vi "VisualizePPS2.vi"() -> ()   [LabVIEW 2018, in "Visualization.lvlib" / "VisualizeAcPwr.lvclass"]
uses:
  VisualizeAcPwr.lvclass
  <vilib>/event_ctls.llb/usereventprio.ctl
  VisualizeBase/VisualizeBase_class/Requests/clUserEventType.ctl
  <vilib>/Utility/error.llb/Error Cluster From Error Code.vi
  <vilib>/ErrorRing/Error Ring.xnode
  VisualizeBase/VisualizeBase_class/VisualizeBase.lvclass
  <userlib>/NIST/NISTErrorLib/NISTErrorLib.lvlib
  AcPwr/AcPwrModule/AcPwrModule.lvlib
panel:
  out "Incorrect DataType?":bool
  in  "PluginName":string="AcPwr.PPS2"
  out "PacificPower":waveform(dbl)[](graph)=[{"t0"=timestamp(3657294743.1094904 s since 1904-01-01), "dt"=1.0, "Y"=[46.242]}, {"t0"=timestamp(3657294743.1094904 s since 1904-01-01), "dt"=1.0, "Y"=[0.304]}, {"t0"=timestamp(3657294743.1094904 s since 1904-01-01), "dt"=1.0, "Y"=[60.0]}] caption="4140002"
  in  "btnStop":bool
  in  "btnReset":bool
  in  "btnClear":bool
  out "ErrorArray":errorcluster[](array[cluster])
  in  "PlotYAxis":u32[](array[numeric])=[0, 1, 0, 0] max=1
  in  "QueueName":string="PPSVQ"
  # "0=Left Axis and 1=Right Axis"
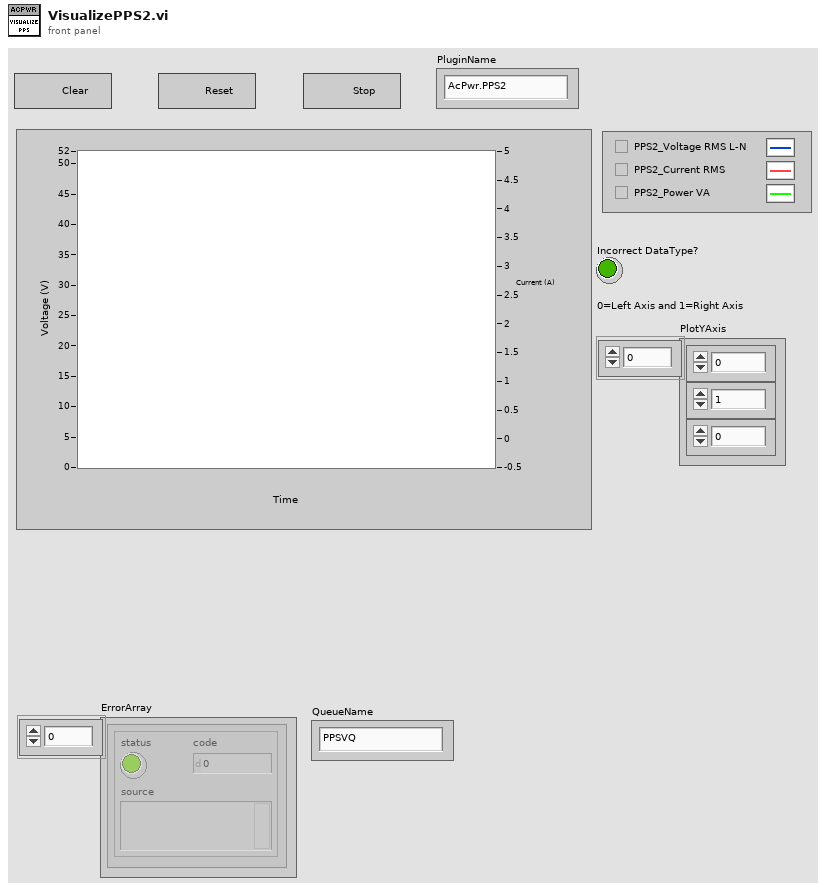
[diagram p1: front panel]
types:
  T1 = typedef "Visualization.lvlib/VisualizeBase.lvclass/clRequestEvents.ctl" = cluster{"StopRequest":refnum<user-event>, "ResetRequest":refnum<user-event>}
  T2 = typedef "AcPwrModule.lvlib/clBroadcastEvents.ctl" = cluster{"DidInit":refnum<user-event>, "StatusUpdate":refnum<user-event>, "ErrorReport":refnum<user-event>, "DidStop":refnum<user-event>, "PathToINI":refnum<user-event>, "Measurements":refnum<user-event>, "LoadConfigFile":refnum<user-event>, "GetSettings":refnum<user-event>, "SetSettings":refnum<user-event>, "GetType&ID":refnum<user-event>, "GotSettings":refnum<user-event>}
  T3 = typedef "Visualization.lvlib/VisualizeBase.lvclass/clUserEventType.ctl" = cluster{"BusIndex":i8, "Data":variant}
  T4 = typedef "usereventprio.ctl" = enum32{"high priority", "normal priority"}
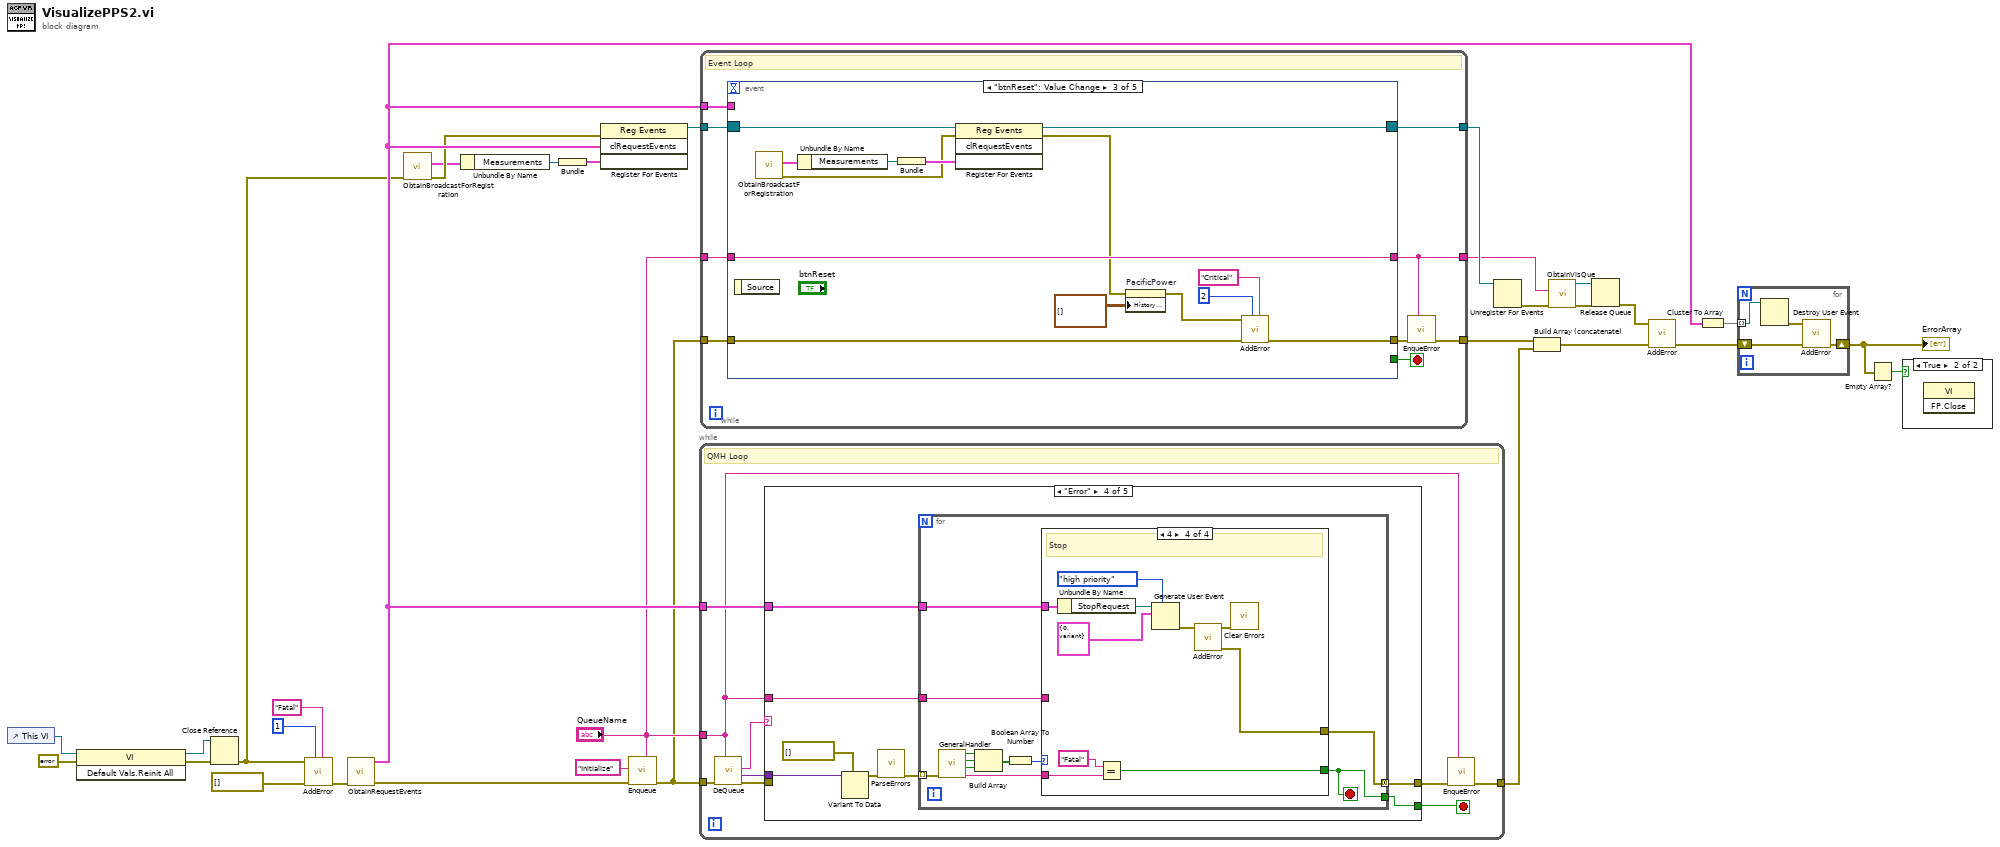
[diagram p0: block diagram]
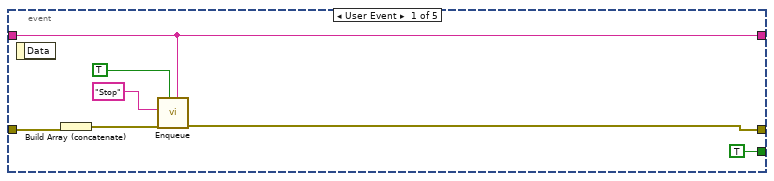
[diagram p2: hidden frame]
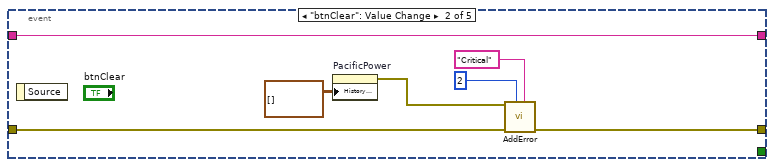
[diagram p3: hidden frame]
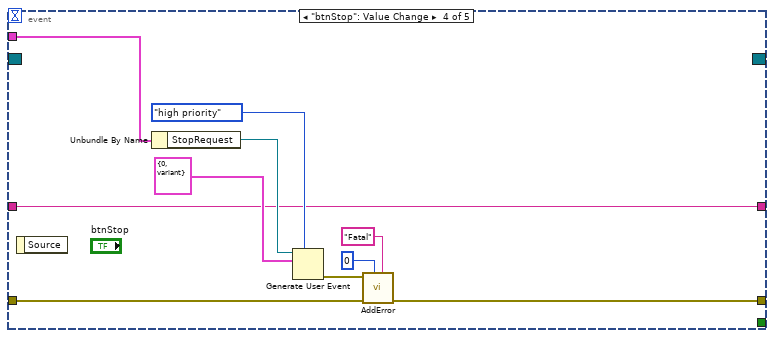
[diagram p4: hidden frame]
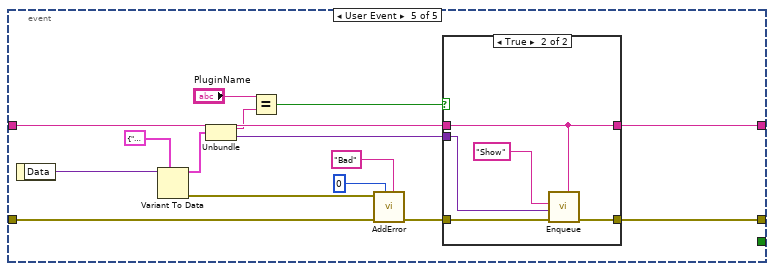
[diagram p5: hidden frame]
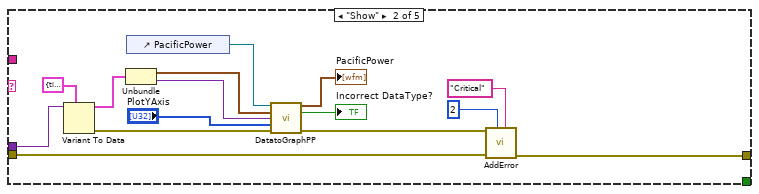
[diagram p8: hidden frame]
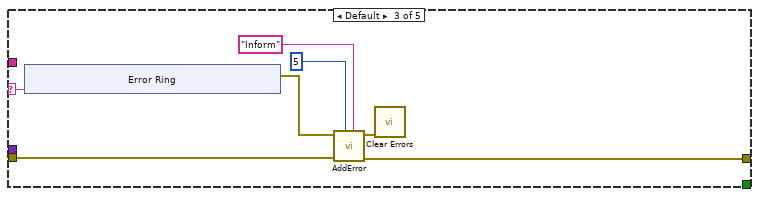
[diagram p9: hidden frame]
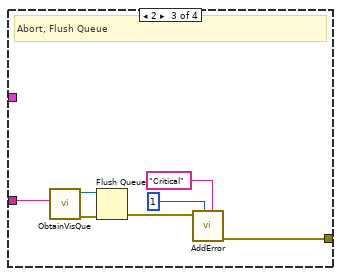
[diagram p12: hidden frame]
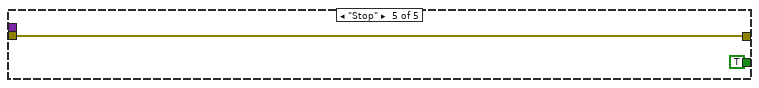
[diagram p13: hidden frame]
diagram:
  n1 = control-ref of="This VI"() -> (w14:refnum<vi>)
  n2 = invoke class="VI" method="Default Vals.Reinit All"(reference=w14, error in=errorcluster {"status"=FALSE, "code"=0, "source"=""} ("error in (no error)")) -> (reference out=w11:refnum<vi>, error out=w12:errorcluster)  [unwired: 1 in, 1 out]
  n3 = Close Reference(reference=w11, error in (no error)=w12) -> (error out=w10:errorcluster)
  n4 = call <userlib>:"AddError.vi"("Severity"="Fatal" ("String"), "Priority"=u8 1, "ErrorArray"=errorcluster[] [], "error in (no error)"=w10) -> ("ErrorArray"=w30:errorcluster[])  [unwired: 6 in, 1 out]
  n5 = call "ObtainRequestEvents.vi"("Error"=w30) -> ("Error"=w15:errorcluster[], "clRequestEvents"=w19:T1)  [unwired: 9 in]
  n6 = call "ObtainBroadcastForRegistration.vi"("error in (no error)"=w10) -> ("error out"=w9:errorcluster, "clBroadcastEvents"=w8:T2)  [unwired: 9 in]
  n7 = Unbundle By Name(w8) -> ("Measurements"=w17:refnum<user-event>)
  n8 = Bundle("Measurements"=w17) -> (w16:cluster{"Measurements":refnum<user-event>})  [unwired: 1 in]
  n9 = register-events(error in=w9, w19, w16) -> (reference out=w31:refnum<event-registration>)  [unwired: 1 in, 1 out]
  n10 = call "Enqueue.vi"("QueName"="QueueName", "Error"=w15, "Message"="Initialize") -> ("Error"=w2:errorcluster[])  [unwired: 8 in]
  n11 = while {
    tunnel: w2 -> [w41]
    tunnel: [w35] -> w26
    tunnel: "QueueName" -> [w33]
    tunnel: w19 -> [w34]
    stop <- w36 stop-if-true
    # "QMH Loop"
    n12 = call "DeQueue.vi"("QueName"=w33, "Error"=w41) -> ("Error"=w38:errorcluster[], "Data"=w39:variant, "Message"=w40:string)  [unwired: 7 in]
    n13 = case shown="\"Error\"" w40 {
      selector: w40 -> [_ _ w64 _ _]
      tunnel: w39 -> [_ w55 _ w79 _]
      tunnel: w38 -> [w42 w52 w62 _ w108]
      tunnel: [w42 w57 w61 w75 w108] -> w37
      tunnel: [_ _ _ w74 TRUE] -> w36
      tunnel: w34 -> [_ _ _ w73 _]
      tunnel: w33 -> [_ _ _ w72 _]
      frame "Initialize" {
      }
      frame "Show" {
        n14 = Variant To Data(type=cluster{timestamp, "Data":variant} {timestamp(0 s since 1904-01-01), "Data"=variant}, Variant=w55) -> (data=w56:cluster{timestamp, "Data":variant}, error out=w47:errorcluster)  [unwired: 1 in]
        n15 = Unbundle(w56) -> (w44:timestamp, "Data"=w43:variant)
        n16 = control-ref of="PacificPower"() -> (w48:refnum<vi>)
        n17 = call "DatatoGraphPP.vi"("PacificPowerChartReference"=w48, "Current time"=w44, "Data"=w43, "PlotYAxis"="PlotYAxis", "error in (no error)"=w47) -> ("Array"=→"PacificPower":waveform(dbl)[], "Incorrect DataType?"=→"Incorrect DataType?":bool, "error out"=w50:errorcluster)  [unwired: 8 in]
        n18 = call <userlib>:"AddError.vi"("Severity"="Critical" ("String"), "Priority"=u8 2, "ErrorArray"=w52, "error in (no error)"=w50) -> ("ErrorArray"=w57:errorcluster[])  [unwired: 6 in, 1 out]
      }
      frame Default {
        n19 = xnode "Error Ring"("parameter 0"=w64) -> ("error out"=w63:errorcluster)
        n20 = call <userlib>:"AddError.vi"("Severity"="Inform" ("String"), "Priority"=u8 5, "ErrorArray"=w62, "error in (no error)"=w63) -> ("ErrorArray"=w61:errorcluster[], "error out"=w60:errorcluster)  [unwired: 6 in]
        n21 = call <vilib>:"Clear Errors.vi"("error in (no error)"=w60) -> ()  [unwired: 5 in, 2 out]
      }
      frame "Error" {
        n22 = Variant To Data(type=errorcluster[] [], Variant=w79) -> (data=w77:errorcluster[])  [unwired: 1 in, 1 out]
        n23 = call <userlib>:"ParseErrors.vi"("ErrorArray"=w77) -> ("ErrorArray"=w76:errorcluster[])  [unwired: 8 in, 2 out]
        n24 = for {
          tunnel: w76 -> [w90] mode=indexing
          tunnel: [w84] -> w75 mode=concatenating
          tunnel: [w82] -> w74
          tunnel: w73 -> [w81]
          tunnel: w72 -> [w80]
          stop <- w82 stop-if-true
          n25 = call <userlib>:"GeneralHandler.vi"("error in (no error)"=w90) -> ("Severity"=w83:string, "Stop"=w87:bool, "Abort"=w88:bool, "Continue"=w89:bool)  [unwired: 7 in]
          n26 = Build Array(w89, w88, w87) -> (w86:bool[])
          n27 = Boolean Array To Number(Boolean array=w86) -> (number=w85:u32)
          n28 = case shown="4" w85 {
            tunnel: [_ _ w95 w106] -> w84
            tunnel: w83 -> [_ _ _ w101]
            tunnel: [_ _ _ w99] -> w82
            tunnel: w81 -> [_ _ _ w98]
            tunnel: w80 -> [_ _ w91 _]
            frame 0, Default {
              # "No Dialog"
            }
            frame 1 {
              # "Continue"
            }
            frame 2 {
              # "Abort, Flush Queue"
              n29 = call "ObtainVisQue.vi"("QueName"=w91) -> ("error out"=w97:errorcluster, "queue out"=w96:refnum<queue>)  [unwired: 9 in]
              n30 = Flush Queue(queue=w96, error in (no error)=w97) -> (error out=w94:errorcluster)  [unwired: 2 out]
              n31 = call <userlib>:"AddError.vi"("Severity"="Critical" ("String"), "Priority"=u8 1, "error in (no error)"=w94) -> ("ErrorArray"=w95:errorcluster[])  [unwired: 7 in, 1 out]
            }
            frame 4 {
              # "Stop"
              n32 = Unbundle By Name(w98) -> ("StopRequest"=w107:refnum<user-event>)
              n33 = Equal?(x="Fatal", y=w101) -> (x = y?=w99:bool)
              n34 = Generate User Event(priority (normal)=usereventprio."high priority", user event=w107, event data cluster=T3 {"BusIndex"=0, "Data"=variant} ("event data")) -> (error out=w105:errorcluster)  [unwired: 1 in, 1 out]
              n35 = call <userlib>:"AddError.vi"("error in (no error)"=w105) -> ("ErrorArray"=w106:errorcluster[], "error out"=w102:errorcluster)  [unwired: 9 in]
              n36 = call <vilib>:"Clear Errors.vi"("error in (no error)"=w102) -> ()  [unwired: 5 in, 2 out]
            }
          }
        }
      }
      frame "Stop" {
      }
    }
    n37 = call "EnqueError.vi"("QueName"=w33, "Error"=w37) -> ("Error"=w35:errorcluster[])  [unwired: 9 in]
  }
  n38 = while {
    tunnel: w31 -> [w118]
    tunnel: [w115] -> w27
    tunnel: [w114] -> w29
    tunnel: w19 -> [w113]
    tunnel: w2 -> [w112]
    tunnel: "QueueName" -> [w111]
    tunnel: [w110] -> w6
    stop <- w117 stop-if-true
    # "Event Loop"
    n39 = event shown="[2] \"btnReset\": Value Change" {
      selector: w118 -> [_ _ w146 _ _]
      dyn-events: [_ _ w145 _ _] -> w114
      timeout: _ -> [_ _ _ _ _]
      tunnel: [TRUE _ _ _ _] -> w117
      tunnel: [w124 w128 w138 w154 w171] -> w116
      tunnel: w113 -> [_ _ _ w149 _]
      tunnel: w112 -> [w121 w129 w139 w147 w160]
      tunnel: w111 -> [w119 w132 w140 w148 w170]
      tunnel: [w119 w132 w140 w148 w161] -> w110
      event User Event {
        n40 = event-data() -> ()  [unwired: 1 in, 1 out]
        n41 = Build Array (concatenate)(w121) -> (w120:errorcluster[])
        n42 = call "Enqueue.vi"("QueName"=w119, "Priority? (F)"=TRUE, "Error"=w120, "Message"="Stop") -> ("Error"=w124:errorcluster[])  [unwired: 7 in]
      }
      event "btnClear": Value Change {
        n43 = event-data() -> ()  [unwired: 1 in, 1 out]
        n44 = property on="PacificPower" class="WFChart (strict)"("History Data"=waveform(dbl)[][] []) -> (error out=w126:errorcluster)  [unwired: 2 in, 1 out]
        n45 = call <userlib>:"AddError.vi"("Severity"="Critical" ("String"), "Priority"=u8 2, "ErrorArray"=w129, "error in (no error)"=w126) -> ("ErrorArray"=w128:errorcluster[])  [unwired: 6 in, 1 out]
      }
      event "btnReset": Value Change {
        n46 = event-data() -> ()  [unwired: 1 in, 1 out]
        n47 = call "ObtainBroadcastForRegistration.vi"() -> ("error out"=w141:errorcluster, "clBroadcastEvents"=w142:T2)  [unwired: 10 in]
        n48 = Unbundle By Name(w142) -> ("Measurements"=w144:refnum<user-event>)
        n49 = Bundle("Measurements"=w144) -> (w143:cluster{"Measurements":refnum<user-event>})  [unwired: 1 in]
        n50 = register-events(reference=w146, error in=w141, w143) -> (reference out=w145:refnum<event-registration>, error out=w134:errorcluster)  [unwired: 1 in]
        n51 = property on="PacificPower" class="WFChart (strict)"(error in=w134, "History Data"=waveform(dbl)[][] []) -> (error out=w133:errorcluster)  [unwired: 1 in, 1 out]
        n52 = call <userlib>:"AddError.vi"("Severity"="Critical" ("String"), "Priority"=u8 2, "ErrorArray"=w139, "error in (no error)"=w133) -> ("ErrorArray"=w138:errorcluster[])  [unwired: 6 in, 1 out]
      }
      event "btnStop": Value Change {
        n53 = event-data() -> ()  [unwired: 1 in, 1 out]
        n54 = Unbundle By Name(w149) -> ("StopRequest"=w155:refnum<user-event>)
        n55 = Generate User Event(priority (normal)=usereventprio."high priority", user event=w155, event data cluster=T3 {"BusIndex"=0, "Data"=variant} ("event data")) -> (error out=w156:errorcluster)  [unwired: 1 in, 1 out]
        n56 = call <userlib>:"AddError.vi"("Severity"="Fatal" ("String"), "Priority"=u8 0, "ErrorArray"=w147, "error in (no error)"=w156) -> ("ErrorArray"=w154:errorcluster[])  [unwired: 6 in, 1 out]
      }
      event User Event {
        n57 = event-data() -> ("Data"=w159:variant)  [unwired: 1 in]
        n58 = Variant To Data(type=cluster{string, "Data":variant} {"", "Data"=variant}, Variant=w159) -> (data=w168:cluster{string, "Data":variant}, error out=w164:errorcluster)  [unwired: 1 in]
        n59 = Unbundle(w168) -> (w167:string, "Data"=w157:variant)
        n60 = Equal?(x="PluginName", y=w167) -> (x = y?=w158:bool)
        n61 = call <userlib>:"AddError.vi"("Severity"="Bad" ("String"), "Priority"=u8 0, "ErrorArray"=w160, "error in (no error)"=w164) -> ("ErrorArray"=w162:errorcluster[])  [unwired: 6 in, 1 out]
        n62 = case shown="True" w158 {
          tunnel: [w173 w177] -> w171
          tunnel: w170 -> [w172 w175]
          tunnel: w162 -> [w173 w176]
          tunnel: [w172 w175] -> w161
          tunnel: w157 -> [_ w174]
          frame False {
          }
          frame True {
            n63 = call "Enqueue.vi"("QueName"=w175, "Error"=w176, "Data"=w174, "Message"="Show") -> ("Error"=w177:errorcluster[])  [unwired: 7 in]
          }
        }
      }
    }
    n64 = call "EnqueError.vi"("QueName"=w110, "Error"=w116) -> ("Error"=w115:errorcluster[])  [unwired: 9 in]
  }
  n65 = Unregister For Events(event registration refnum=w29) -> (error out=w25:errorcluster)  [unwired: 1 in]
  n66 = Build Array (concatenate)(w27, w26) -> (w24:errorcluster[])
  n67 = call "ObtainVisQue.vi"("error in (no error)"=w25, "QueName"=w6) -> ("error out"=w23:errorcluster, "queue out"=w22:refnum<queue>)  [unwired: 8 in]
  n68 = Release Queue(queue=w22, error in (no error)=w23) -> (error out=w21:errorcluster)  [unwired: 1 in, 2 out]
  n69 = call <userlib>:"AddError.vi"("ErrorArray"=w24, "error in (no error)"=w21) -> ("ErrorArray"=w20:errorcluster[])  [unwired: 8 in, 1 out]
  n70 = Cluster To Array(cluster=w19) -> (array=w28:refnum<user-event>[])
  n71 = for {
    tunnel: w28 -> [w182] mode=indexing
    shift-right: [w181] -> w1
    shift-left: w20 -> [w180]
    n72 = Destroy User Event(user event=w182) -> (error out=w179:errorcluster)  [unwired: 1 in]
    n73 = call <userlib>:"AddError.vi"("ErrorArray"=w180, "error in (no error)"=w179) -> ("ErrorArray"=w181:errorcluster[])  [unwired: 8 in, 1 out]
  }
  "ErrorArray" <- w1
  n74 = Empty Array?(array=w1) -> (empty?=w18:bool)
  n75 = case shown="True" w18 {
    frame False {
    }
    frame True {
      n76 = invoke class="VI" method="FP.Close"() -> ()  [unwired: 3 in, 3 out]
    }
  }
